vi "PL_Global.vi"() -> ()   [LabVIEW 2020]
panel:
  in  "Cluster":cluster{"NAMES":string[], "ID":dbl[]}
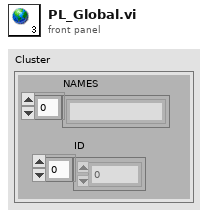
[diagram p1: front panel]
diagram:
